vi "KM_Primer.vi"(1 "С":bool, 2 "Reset":bool, 3 "Cluster":T2) -> (0 "Q":T1)   [LabVIEW 2012]
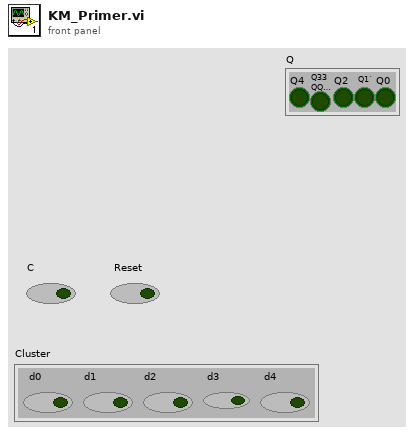
[diagram p1: front panel]
types:
  T1 = cluster{"Q4":bool, "Q33QQq3Q3Q3Q3Q3Q3Q3Q":bool, "Q2":bool, "Q1`":bool, "Q0":bool}
  T2 = cluster{"d0":bool, "d1":bool, "d2":bool, " d3":bool, " d4":bool}
  T3 = cluster{"q":bool, "q":bool, "q":bool, "q":bool, "q":bool}
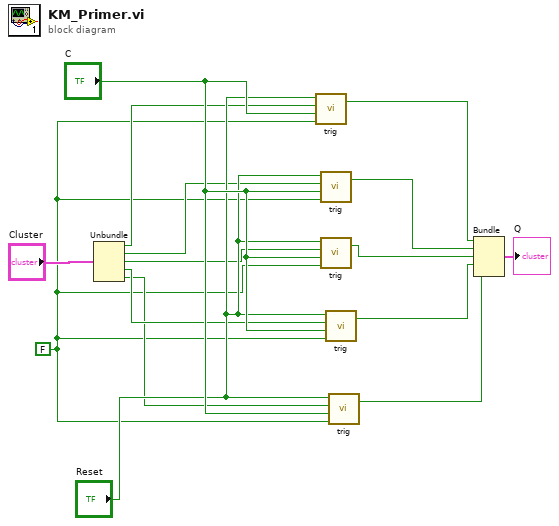
[diagram p0: block diagram]
diagram:
  w7 = FALSE
  n1 = Unbundle("Cluster") -> ("d0"=w12:bool, "d1"=w11:bool, "d2"=w10:bool, "d3"=w9:bool, "d4"=w8:bool)
  n2 = call "trig.vi"("s"=w7, "c"="С", "d"=w12, "r"="Reset") -> ("q"=w6:bool)  [unwired: 1 out]
  n3 = call "trig.vi"("s"=w7, "c"="С", "d"=w11, "r"="Reset") -> ("q"=w5:bool)  [unwired: 1 out]
  n4 = call "trig.vi"("s"=w7, "c"="С", "d"=w10, "r"="Reset") -> ("q"=w4:bool)  [unwired: 1 out]
  n5 = call "trig.vi"("s"=w7, "c"="С", "d"=w9, "r"="Reset") -> ("q"=w3:bool)  [unwired: 1 out]
  n6 = call "trig.vi"("s"=w7, "c"="С", "d"=w8, "r"="Reset") -> ("q"=w2:bool)  [unwired: 1 out]
  n7 = Bundle("q"=w6, "q"=w5, "q"=w4, "q"=w3, "q"=w2) -> (→"Q":T3)  [unwired: 1 in]
